vi "preset pos Read.vi"(4 "error in (no error)":errorcluster, 6 "Container State":T3, 7 "Display State In":T1={"Cells_VD2"=enum."5", "position"=0.0, "DS param"={"Domain name"="manip", "experiment"="VD2", "Device Server name"="DLs_VD2", "DL param"={"real pos"=-137.0, "max"=-30.0, "min"=120.0}, "preset pos"=[]}, "event"=refnum}) -> (0 "error out":errorcluster, 2 "Value":dbl[](array[numeric]), 3 "Display State Out":T1={"Cells_VD2"=enum."5", "position"=0.0, "DS param"={"Domain name"="manip", "experiment"="VD2", "Device Server name"="DLs_VD2", "DL param"={"real pos"=-137.0, "max"=-30.0, "min"=120.0}, "preset pos"=[]}, "event"=refnum})   [LabVIEW 2020, in "OWIS_DLs_h.xctl"]
uses:
  OWIS_DLs_h.xctl
  <vilib>/_xctls/Container State.ctl
  stateDL.ctl
  controls/CellsSDI.ctl
  controls/CellBoolean.ctl
  <vilib>/_xctls/XControlSupport.lvlib
panel:
  # "Replace the Value Indicator below with an Indicator of desired type.\nDo not remove this Indicator or the others from the connector pane. \nDo not change the connector pane pattern.\nThe Value Indicator should always be the second terminal from top on the output side in the connector pane."
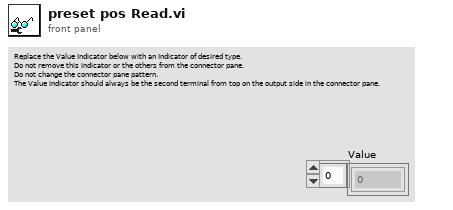
[diagram p1: front panel]
types:
  T1 = typedef "OWIS_DLs_h.xctl/stateDL.ctl" = cluster{"Cells_VD2":T2, "position":dbl, "DS param":cluster{"Domain name":string, "experiment":string, "Device Server name":string, "DL param":cluster{"real pos":dbl, "max":dbl, "min":dbl}, "preset pos":dbl[]}, "event":refnum<user-event>}
  T2 = typedef "CellsSDI.ctl" = enum32{"5", "4", "3", "2", "1", "L"}
  T3 = typedef "XControlSupport.lvlib/Container State.ctl" = cluster{"Indicator?":bool, "Run Mode?":bool, " Refnum":refnum<vi>}
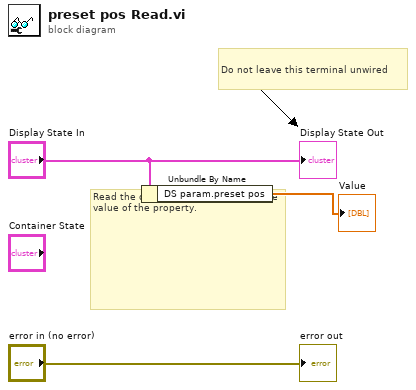
[diagram p0: block diagram]
diagram:
  # "Do not leave this terminal unwired"
  # "Read the display state and update the value of the property."
  n1 = Unbundle By Name("Display State In") -> ("DS param.preset pos"=→"Value":dbl[])
  "error out" <- "error in (no error)"
  "Display State Out" <- "Display State In"
